vi "LOAD CELL READ.vi"(8 "error in (no error)":errorcluster, 11 "main ref":T1) -> (0 "error out":errorcluster)   [LabVIEW 2025]
uses:
  controls/LAB-IQ UI Data.ctl
  Traction Loop/Traction Receipe Enum.ctl
  v05/LOAD CELL CODE/New Logic/Load cell Enum.ctl
  <vilib>/Analysis/baseanly.llb/Mean (DBL).vi
  <vilib>/Analysis/5stat.llb/RMS (DBL).vi
  <vilib>/Analysis/Matrix/Numeric/Conversions/Array To Matrix - RA.vi
  <vilib>/Analysis/Matrix/Numeric/Conversions/Matrix To Array - RM.vi
  <vilib>/Analysis/NI_AALBase.lvlib
  <vilib>/ptbypt/NI_PtbyPt.lvlib
  <vilib>/Analysis/NI_AALPro.lvlib
  <vilib>/Analysis/Matrix/NI_Matrix.lvlib
panel:
  out "Fload 3":dbl
  out "Fload 2":dbl
  out "Fload":dbl
  out "Friction":dbl
  out "Load Temp":dbl
  out "Zload":dbl
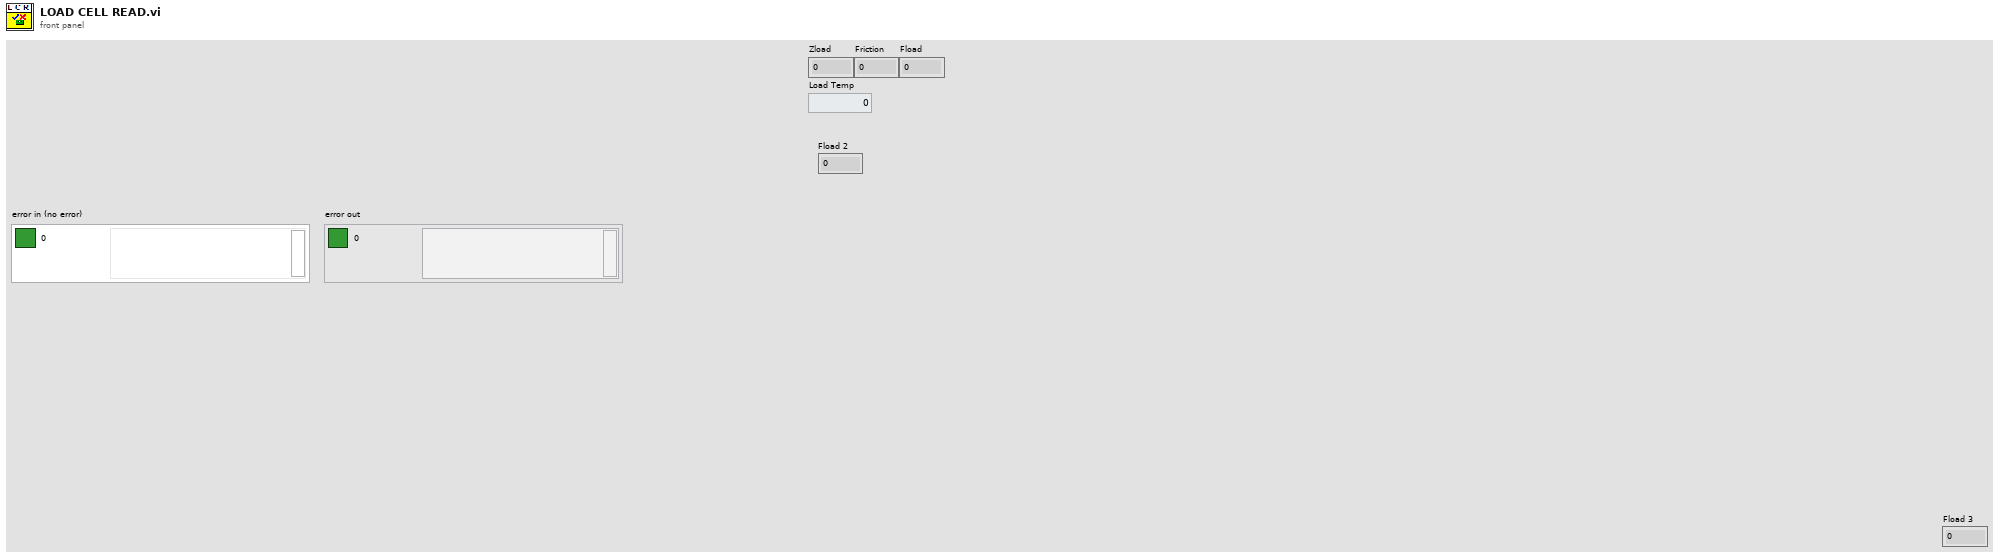
[diagram p1: front panel]
types:
  T1 = typedef "LAB-IQ UI Data.ctl" = cluster{"Main Home Screen":cluster{"GUI":refnum<vi>, "Platform Settings":refnum<vi>, "Configure":refnum<vi>, "Home":refnum<vi>, "EXIT":refnum<vi>, "service 2":refnum<vi>, "MainPage":refnum<vi>, "Analysis":refnum<vi>}, "Platform Settings":cluster{"mm/s  Surge":refnum<vi>, "Drive Error":refnum<vi>, "Disable Axis Jog Soft Limits":refnum<vi>, "mm/s  Sway":refnum<vi>, "Sway and Surge COM Status":refnum<vi>, "Heave COM Status":refnum<vi>, "Enable Platform":refnum<vi>, "Surge Forward Main":refnum<vi>, "Sway Right Main":refnum<vi>, "Sway Left Main":refnum<vi>, "Heave Down Main":refnum<vi>, "Heave Up main":refnum<vi>, "mm/s Heave":refnum<vi>, "mm/sec":refnum<vi>, "mm":refnum<vi>, "Surge Backward Main":refnum<vi>}, "Analysis Screen":cluster{"Analysis Home":refnum<vi>, "Surface Analysis":refnum<vi>, "Imaging":refnum<vi>, "Image Analysis":refnum<vi>, "Post Analysis":refnum<vi>}, "Config Screen":cluster{"Select Load Head":refnum<vi>, "Notes :":refnum<vi>, "FILE":refnum<vi>, "Sample ID :":refnum<vi>, "Operator ID :":refnum<vi>, "Operator Name :":refnum<vi>, "Auto":refnum<vi>}, "Motion Module":cluster{"zNL":refnum<vi>, "NL disp":refnum<vi>, "Rotary Tab":refnum<vi>, "Motion Direction:  3":refnum<vi>, "E.Velocity 2":refnum<vi>, "e.v/ssr 2":refnum<vi>, "Enter Fixed E.Velocity 2":refnum<vi>, "Enter Final SRR 2":refnum<vi>, "Enter initial SRR 2":refnum<vi>, "Enter Fixed SRR 2":refnum<vi>, "Enter the Final E.Velocity (m/s) 2":refnum<vi>, "Enter initial E.Velocity (m/s) 2":refnum<vi>, "Final Speed (RPM) 3":refnum<vi>, "Initial Speed (RPM) 2":refnum<vi>, "Enter the Final Velocity (m/s) 3":refnum<vi>, "Enter initial Velocity (m/s)  3":refnum<vi>, "Ramp Up 2":refnum<vi>, "TEST SELECTION":refnum<vi>, "SPEED SELECTION : ":refnum<vi>, "Angular Oscillation Set":refnum<vi>, "Traction":refnum<vi>, "Step Speed":refnum<vi>, "StepTable For Load-Speed":refnum<vi>, "StepTable For Speed":refnum<vi>, "Surge Forward MM":refnum<vi>, "Surge Backward MM":refnum<vi>, "M3 Image":refnum<vi>, "String 39":refnum<vi>, "Sway Left MM":refnum<vi>, "Sway Right MM":refnum<vi>, "Disable Axis Jog Soft Limits":refnum<vi>, "mm":refnum<vi>, "Heave Down MM":refnum<vi>, "Heave Up MM":refnum<vi>, "Wear Track Diameter (mm)":refnum<vi>, "Set WTD":refnum<vi>, "HomeScratch":refnum<vi>, "HomeRot":refnum<vi>, "PlaceModule":refnum<vi>, "Enter the Angle (Deg)":refnum<vi>, "Enter the Frequency (Hz)":refnum<vi>, "Motion Mode:":refnum<vi>, "LR Sway":refnum<vi>, "Rot Hor":refnum<vi>, "Scratch":refnum<vi>, "LR Cam":refnum<vi>, "MMBack":refnum<vi>, "MMNext":refnum<vi>, "Rot Ver":refnum<vi>, "Rotary Module Selection":refnum<vi>, "calculate rotary":refnum<vi>, "SPEED SELECTION : rotary":refnum<vi>, "Import 2":refnum<vi>, "Save 2":refnum<vi>, "File Path :  2":refnum<vi>, "String 45":refnum<vi>, "StepTable For Speed 3":refnum<vi>, "Enter the Speed(mm/sec)":refnum<vi>, "Enter the Speed(RPM)":refnum<vi>, "Enter Scratch Speed (mm/s):":refnum<vi>, "SwaySpeed Set":refnum<vi>, "Scartch Offset":refnum<vi>, "Motion type:":refnum<vi>, "HomeScratch 2":refnum<vi>, "Enter Scratch length (mm):":refnum<vi>, "Wear Track Diameter":refnum<vi>, "Rotary Speed Exced":refnum<vi>, "Scratch Mode":refnum<vi>, "No of Scratch":refnum<vi>}, "Environmental control":cluster{"Humidity  Status  3":refnum<vi>, "Low Temp  Status  2":refnum<vi>, "TK4 status 2":refnum<vi>, "Stage Temperature":refnum<vi>, "Sample Temperature":refnum<vi>, "Humidity (Amb)":refnum<vi>, "Clear List":refnum<vi>, "Add to list":refnum<vi>, "Wear":refnum<vi>, "Vibration":refnum<vi>, "Humidity (Chamber)":refnum<vi>, "Temperature (Chamber)":refnum<vi>, "ECR ":refnum<vi>, "Temperature (Amb)":refnum<vi>, "Microphone":refnum<vi>, "Acoustic Emission 3":refnum<vi>, "SNext":refnum<vi>, "APBack":refnum<vi>, "Enter the Temperature (°C):":refnum<vi>, "Enter the Stage \nTemperature (°C):":refnum<vi>, "Enter the Humidity (%Rh):":refnum<vi>, "Low Temp":refnum<vi>, "High Temp":refnum<vi>, "Humidity":refnum<vi>, "Sensors Picked":refnum<vi>}, "About Screen":cluster{"Password":refnum<vi>, "Home Service":refnum<vi>, "Advanced Setting":refnum<vi>, "About Tab":refnum<vi>, "ECR Port:":refnum<vi>, "Ramp Port:":refnum<vi>, "Installation/Replacement completed":refnum<vi>, "Loahead":refnum<vi>, "Heave and Surge COM Port:":refnum<vi>, "Sway COM Port:":refnum<vi>, "Temp Modbus:":refnum<vi>, "Humidity Port:":refnum<vi>, "Edit Gain Constants":refnum<vi>, "Save Gain Constants":refnum<vi>}, "Main Screen":cluster{"Main Screen Tab":refnum<vi>, "Angle and Frequency":refnum<vi>, "Stroke (mm)":refnum<vi>, "Angle (Deg)":refnum<vi>, "Main Speed Tab":refnum<vi>, "MTM MOTOR DISPLAY":refnum<vi>, "Disc Speed (m/sec)":refnum<vi>, "Ball Speed (m/sec)":refnum<vi>, "Disc Speed (RPM)":refnum<vi>, "Ball Speed (RPM)":refnum<vi>, "SPEED TAB":refnum<vi>, "Speed (m/sec)":refnum<vi>, "Set Speed (m/sec)":refnum<vi>, "Speed (RPM)":refnum<vi>, "Set Speed":refnum<vi>, "Time Tab":refnum<vi>, "Time ( HH:MM:SS ) 2":refnum<vi>, "Test Duration":refnum<vi>, "Test Duration 4":refnum<vi>, "TEST CYCLE":refnum<vi>, "TOTAL CYCLES":refnum<vi>, "Set Load (N)":refnum<vi>, "Temp Tabs":refnum<vi>, "Heater":refnum<vi>, "TK4 status":refnum<vi>, "ChamberTemp":refnum<vi>, "SetTmp":refnum<vi>, "Controller  Status":refnum<vi>, "ChamberTemp 2":refnum<vi>, "SetTmp 2":refnum<vi>, "Controller  Status 2":refnum<vi>, "ChamberTemp 3":refnum<vi>, "SetTmp 3":refnum<vi>, "Cooling":refnum<vi>, "Load Communication":refnum<vi>, "Ambient \nTemperature":refnum<vi>, "HumCOMStatus":refnum<vi>, "Ambient\n Humidity":refnum<vi>, "Freq (Hz)":refnum<vi>, "Load En":refnum<vi>, "NLt":refnum<vi>, "zNL 2":refnum<vi>, "Humidity On":refnum<vi>, "humidity disp":refnum<vi>, "Set Humidity":refnum<vi>, "NL disp 2":refnum<vi>, "Humidity On 2":refnum<vi>, "humidity disp 2":refnum<vi>, "Set Humidity 2":refnum<vi>, "NL disp 3":refnum<vi>, "AppLoadSeq scratch":refnum<vi>, "Stop Scratch":refnum<vi>, "ClrLog":refnum<vi>, "Trip Log":refnum<vi>, "STOP":refnum<vi>, "Start Test":refnum<vi>, "Test status":refnum<vi>, "AR Led":refnum<vi>, "Data":refnum<vi>, "Health":refnum<vi>, "Sway COM Status":refnum<vi>, "Heave COM Status":refnum<vi>, "Grp Tab":refnum<vi>, "Sub Graph":refnum<vi>, "SD (mm)":refnum<vi>, "Siliding distance Reset Graph":refnum<vi>, "SDGp":refnum<vi>, "Humidity Reset Graph":refnum<vi>, "HumrGp":refnum<vi>, "Acoustic Emission (mV)":refnum<vi>, "Aqucostic Reset Graph":refnum<vi>, "gACQUOS":refnum<vi>, "ECR RESET":refnum<vi>, "ECR":refnum<vi>, "Temperature Reset":refnum<vi>, "Acoustic Emission (mV) 2":refnum<vi>, "Aqucostic Reset Graph 2":refnum<vi>, "gACQUOS 2":refnum<vi>, "ECR RESET 2":refnum<vi>, "ECR 2":refnum<vi>, "Temperature Reset 2":refnum<vi>, "Temperature (deg c)":refnum<vi>, "Speed Reset Graph":refnum<vi>, "Speed Tab":refnum<vi>, "MTM DISC  SPEED":refnum<vi>, "MTM BALL SPEED":refnum<vi>, "speed mm/sec":refnum<vi>, "Hymidity":refnum<vi>, "Humidity Disable trip":refnum<vi>, "CoF Trip  2":refnum<vi>, "Depth Trip":refnum<vi>, "Weart Deapth":refnum<vi>, "Depth Reset Graph":refnum<vi>, "Weart":refnum<vi>, "Depthz":refnum<vi>, "Depth (µm)":refnum<vi>, "WearGp":refnum<vi>, "NL Trip 2":refnum<vi>, "Load pid":refnum<vi>, "Load Disable Trip":refnum<vi>, "Load Reset Graph":refnum<vi>, "NL Display 4":refnum<vi>, "Main Chart 3":refnum<vi>, "BACK":refnum<vi>, "Depth Trip 2":refnum<vi>, "COF TRIP ":refnum<vi>, "Friction Force (N)":refnum<vi>, "FF Reset Graph":refnum<vi>, "FF Disable Trip":refnum<vi>, "FF TRIP":refnum<vi>, "COF Disable Trip":refnum<vi>, "COF Reset Graph":refnum<vi>, "Start Test Temp":refnum<vi>, "zFF":refnum<vi>, "Friction Force (N) Graph":refnum<vi>, "Coefficient of Friction":refnum<vi>, "Scratch Start Test":refnum<vi>, "FF Tab":refnum<vi>, "Cyclic Friction Force (N)":refnum<vi>, "CZ FF":refnum<vi>, "Cyclic Friction Force (N) Graph":refnum<vi>, "Cyclic Coefficient of Friction":refnum<vi>, "Cyclic FF TRIP":refnum<vi>, "Cyclic FF Disable Trip":refnum<vi>, "cyclic COF Disable Trip":refnum<vi>, "cyclic COF TRIP":refnum<vi>, "cyclic COF Reset Graph":refnum<vi>, "Cyclic FF Reset Graph":refnum<vi>, "Test Trip":refnum<vi>, "Multi Scratch Pass":refnum<vi>, "Scratch Start Recording":refnum<vi>}, "Loading":cluster{"Indentation":refnum<vi>, "Reference Sample":refnum<vi>, "Load Cell Communication Slide":refnum<vi>, "com 3":refnum<vi>, "com":refnum<vi>, "DecaForce COM Status":refnum<vi>, "Update":refnum<vi>, "Clear 3":refnum<vi>, "seq":refnum<vi>, "Stribeck table":refnum<vi>, "Stribeck Table  For loading":refnum<vi>, "Loading Mode":refnum<vi>, "Enter the Final Load (N)":refnum<vi>, "Enter the CoF Trip":refnum<vi>, "Enter the Friction Force Trip":refnum<vi>, "Enter the Normal load Trip":refnum<vi>, "Enter the Load  (N)":refnum<vi>, "KiloForce":refnum<vi>, "DecaForce ":refnum<vi>, "MicroForce":refnum<vi>, "LHBack":refnum<vi>, "LHNext":refnum<vi>, "Enter the Loading Rate (N/min)":refnum<vi>, "Message":refnum<vi>, "Warning 2":refnum<vi>, "SSP 0.75":refnum<vi>, "SSP 0.5":refnum<vi>, "SSP 0.3":refnum<vi>, "Warning":refnum<vi>, "gui GIF":refnum<vi>, "Communication is established":refnum<vi>, "AppLoad 4":refnum<vi>, "Multipoint":refnum<vi>, "Load Selection":refnum<vi>}, "PID":cluster{"Ramp":refnum<vi>, "Vertical load (N)":refnum<vi>, "apply load":refnum<vi>, "apply load 2":refnum<vi>, "Enter ByPass Load":refnum<vi>, "Bypass Load":refnum<vi>, "gFF Rot":refnum<vi>}, "Config Parameters":cluster{"Tab Control 3":refnum<vi>, "Tab Control 19":refnum<vi>, "SAMPLES":refnum<vi>, "Re-initilaize":refnum<vi>, "Filter ON/OFF":refnum<vi>, "TracHomeSurgeOffsetCounts 10MM":refnum<vi>, "TracHomeSwayOffsetCounts 10MM":refnum<vi>, "Acoustic Emission:":refnum<vi>, "Apply Filter (FF)":refnum<vi>, "Filter% 2":refnum<vi>, "Apply Filter (Load)":refnum<vi>, "Filter% ":refnum<vi>, "Sway distance (mm)":refnum<vi>, "Surge distance (mm)":refnum<vi>, "DataSavingLoopDelay(ms)":refnum<vi>, "SAVE 2":refnum<vi>, "Enter Distance":refnum<vi>, "Sway Counts:":refnum<vi>, "Distance (mm): 3":refnum<vi>, "Surge Counts:":refnum<vi>, "Distance (mm): 2":refnum<vi>, "Distance (mm):":refnum<vi>, "Heave Counts:":refnum<vi>, "LRMHomeSurgeOffsetCounts":refnum<vi>, "LRMHomeSwayOffsetCounts":refnum<vi>, "TracHomeSurgeOffsetCounts 20MM":refnum<vi>, "TracHomeSwayOffsetCounts 20MM":refnum<vi>, "RotHomeSwayOffsetCounts":refnum<vi>, "RotHomeSurgeOffsetCounts":refnum<vi>, "Heave distance":refnum<vi>, "Zmm":refnum<vi>, "Heave Pulses/mm":refnum<vi>, "Surge Pulses/mm":refnum<vi>, "Sway Pulses/mm":refnum<vi>, "Heave Pitch":refnum<vi>, "Surge Pitch":refnum<vi>, "Sway Pitch":refnum<vi>, "Heave PPR":refnum<vi>, "Surge PPR":refnum<vi>, "Sway PPR":refnum<vi>, "Tab Control 5":refnum<vi>, "Tab Control 14":refnum<vi>, "Tab Control 26":refnum<vi>, "AE":refnum<vi>, "Heave Loop Delay":refnum<vi>, "Heave PID Speed":refnum<vi>, "Surge Jog Speed":refnum<vi>, "Heave Jog Speed":refnum<vi>, "Sway Loop Delay":refnum<vi>, "Sway PID Speed":refnum<vi>, "Sway Jog Speed":refnum<vi>, "DEPTH TRIP VALUE":refnum<vi>, "LOAD TRIP VALUE":refnum<vi>, "DEPTH TRIP   ENABLE":refnum<vi>, "LOAD TRIP  ENABLE":refnum<vi>, "CYCLIC FF TRIP VALUE":refnum<vi>, "FF TRIP VALUE":refnum<vi>, "CYCLIC CoF TRIP VALUE":refnum<vi>, "COF TRIP VALUE":refnum<vi>, "CYCLIC COF TRIP  ENABLE":refnum<vi>, "CYCLIC FF TRIP  ENABLE":refnum<vi>, "FF TRIP  ENABLE":refnum<vi>, "COF TRIP  ENABLE":refnum<vi>, "JOG TRIP LOAD VALUE (N)":refnum<vi>, "Rotary Vertical":refnum<vi>, "Traction":refnum<vi>, "Scratch":refnum<vi>, "LRM CAM":refnum<vi>, "Sway LRM":refnum<vi>, "Rotary Horizontal":refnum<vi>}, "Loading Com Port":cluster{"ClearAll":refnum<vi>, "Mz(Nm)":refnum<vi>, "My(Nm)":refnum<vi>, "Mx(Nm)":refnum<vi>, "Save Dwell":refnum<vi>, "Acq Delay (ms)":refnum<vi>, "Burst Delay (ms)":refnum<vi>, "model":refnum<vi>, "SN":refnum<vi>, "FFx(N)":refnum<vi>, "Sensor IP":refnum<vi>, "Port":refnum<vi>, "FFy(N)":refnum<vi>, "Load(N)":refnum<vi>, "delete Handle":refnum<vi>, "Create Handle":refnum<vi>, "ft_data":refnum<vi>, "ft_range":refnum<vi>, "ft_data 2":refnum<vi>, "stop 6":refnum<vi>, "running_flag":refnum<vi>, "ft_udp_handle":refnum<vi>, "get-data-return":refnum<vi>, "get-range-return":refnum<vi>, "zero-return":refnum<vi>, "filter-return":refnum<vi>, "initial-return":refnum<vi>, "deleteHandle-result":refnum<vi>, "Load Cell Temp":refnum<vi>, "Load Cell":refnum<vi>, "ZeroAll":refnum<vi>, "FORCE (N)":refnum<vi>, "TORQUE (N-m)":refnum<vi>, "Load Cell Link":refnum<vi>}, "Heave AND Surge":cluster{"SURGE POSE":refnum<vi>, "error out Read":refnum<vi>, "HEAVE POSE":refnum<vi>, "State":refnum<vi>, "Homed":refnum<vi>, "Sequence ID":refnum<vi>, "error out Write":refnum<vi>, "faultCode":refnum<vi>, "Ack ID":refnum<vi>, "SPEED":refnum<vi>, "Distance":refnum<vi>, "Mode Command":refnum<vi>, "Heave and Surge Read":refnum<vi>, "Read Heave Temp":refnum<vi>, "Spare 15":refnum<vi>, "Spare 14":refnum<vi>, "Spare 13":refnum<vi>, "Spare 12":refnum<vi>, "Spare 11":refnum<vi>, "Spare 10":refnum<vi>, "Spare 9":refnum<vi>, "Spare 8":refnum<vi>, "Spare 7":refnum<vi>, "Spare 4":refnum<vi>, "Spare 3":refnum<vi>, "Spare 2":refnum<vi>, "Humidity":refnum<vi>, "Temp":refnum<vi>, "Node Id":refnum<vi>, "Spare 1":refnum<vi>, "SPARE 4":refnum<vi>, "SPARE 3":refnum<vi>, "SPARE 2":refnum<vi>, "SPARE 1":refnum<vi>, "fwMajor":refnum<vi>, "fwMinor":refnum<vi>, "Manual Write":refnum<vi>, "Heave and Surge Write":refnum<vi>, "SPARE 5":refnum<vi>, "Reserved ":refnum<vi>, "SPARE 8":refnum<vi>, "SPARE 6":refnum<vi>, "SPARE 7":refnum<vi>, "SPARE 17":refnum<vi>, "SPARE 16":refnum<vi>, "SPARE 15":refnum<vi>, "SPARE 14":refnum<vi>, "SPARE 13":refnum<vi>, "SPARE 12":refnum<vi>, "SPARE 11":refnum<vi>, "SPARE 10":refnum<vi>, "SPARE 9":refnum<vi>, "System UPTIME":refnum<vi>, "Missed Packets":refnum<vi>, "faultCode Surge Right":refnum<vi>, "faultCode Surge Left":refnum<vi>, "faultCode Heave":refnum<vi>, "UPLINK HEAVE":refnum<vi>, "DOWNLINK HEAVE":refnum<vi>}, "New PID LOGIC":cluster{"Fine Tune Zone":refnum<vi>, "PID SDelay":refnum<vi>, "Max_pos_limit":refnum<vi>, "Min_pos_limit":refnum<vi>, "i_limit":refnum<vi>, "pct_scale":refnum<vi>, "Deadband":refnum<vi>, "Kd":refnum<vi>, "Ki":refnum<vi>, "Kp":refnum<vi>, "Current Position":refnum<vi>, "Set Load":refnum<vi>, "Current Load":refnum<vi>, "Pulse delta":refnum<vi>, "Init Step":refnum<vi>, "Max Step Linit":refnum<vi>, "min_deadband_floor":refnum<vi>, "dynamic_spindle_noise_scalar":refnum<vi>, "min_finetune_floor":refnum<vi>, "filter_alpha":refnum<vi>, "PID":refnum<vi>}, "SWAY ":cluster{"fwMajor":refnum<vi>, "Homed":refnum<vi>, "Rotary POSE":refnum<vi>, "State":refnum<vi>, "SWAY POSE":refnum<vi>, "Ack ID":refnum<vi>, "faultCode":refnum<vi>, "Node Id":refnum<vi>, "fwMinor":refnum<vi>, "Spare 6":refnum<vi>, "Spare 5":refnum<vi>, "Spare 4":refnum<vi>, "Spare 3":refnum<vi>, "Spare 2":refnum<vi>, "Spare 1":refnum<vi>, "Spare 7":refnum<vi>, "SPARE  5":refnum<vi>, "error out Write  SWAY ":refnum<vi>, "error out Read SWAY ":refnum<vi>, "Manual Write SWAY ":refnum<vi>, "SWAY WRITE":refnum<vi>, "SPARE  4":refnum<vi>, "SPARE  3":refnum<vi>, "SPARE 2":refnum<vi>, "SPARE 1":refnum<vi>, "Spare 15":refnum<vi>, "Spare 14":refnum<vi>, "Spare 13":refnum<vi>, "Spare 12":refnum<vi>, "Spare 11":refnum<vi>, "Spare 9":refnum<vi>, "Spare 8":refnum<vi>, "SPEED":refnum<vi>, "Distance":refnum<vi>, "Mode Command":refnum<vi>, "Sequence ID":refnum<vi>, "SWAY READ":refnum<vi>, "Spare 10":refnum<vi>, "Read SWAY Temp":refnum<vi>, "faultCode Sway ":refnum<vi>, "Missed Packets":refnum<vi>, "System UPTIME sway":refnum<vi>, "SPARE 6":refnum<vi>, "SPARE 7":refnum<vi>, "SPARE 9":refnum<vi>, "SPARE 11":refnum<vi>, "SPARE 10":refnum<vi>, "SPARE 8":refnum<vi>, "SPARE 13":refnum<vi>, "SPARE 12":refnum<vi>, "SPARE 17":refnum<vi>, "SPARE 16":refnum<vi>, "SPARE 15":refnum<vi>, "SPARE 14":refnum<vi>, "Reserved":refnum<vi>, "faultCode Rotary":refnum<vi>, "UPLINK SWAY":refnum<vi>, "DOWNLINK SWAY":refnum<vi>}, "Analysis Screen":cluster{"Analysis Home":refnum<vi>, "Refresh 2":refnum<vi>, "MEAN 4":refnum<vi>, "SD 4":refnum<vi>, "VARIANCE 4":refnum<vi>, "MEAN  3":refnum<vi>, "SD  3":refnum<vi>, "VARIANCE  3":refnum<vi>, "MEAN 2":refnum<vi>, "SD  2":refnum<vi>, "VARIANCE 2":refnum<vi>, "MEAN":refnum<vi>, "SD":refnum<vi>, "VARIANCE":refnum<vi>, "File 4 Discription":refnum<vi>, "OPEN 4":refnum<vi>, "File Name 4":refnum<vi>, "OPEN 3":refnum<vi>, "File 3 Discription":refnum<vi>, "File Name 3":refnum<vi>, "Y-AXIS":refnum<vi>, "X-AXIS":refnum<vi>, "XY Graph":refnum<vi>, "File Name 2":refnum<vi>, "File Name 1":refnum<vi>, "OPEN 2":refnum<vi>, "OPEN 1":refnum<vi>, "File 1 Discription ":refnum<vi>, "File 2 Discription":refnum<vi>, "Export":refnum<vi>, "File Format":refnum<vi>}, "Traction":cluster{"faultCode Traction 2":refnum<vi>, "faultCode Traction 1":refnum<vi>, "Missed Packets":refnum<vi>, "System UPTIME Traction":refnum<vi>, "SPARE 17":refnum<vi>, "SPARE 16":refnum<vi>, "SPARE 15":refnum<vi>, "SPARE 14":refnum<vi>, "SPARE 13":refnum<vi>, "SPARE 12":refnum<vi>, "SPARE 11":refnum<vi>, "SPARE 10":refnum<vi>, "SPARE 9":refnum<vi>, "SPARE 8":refnum<vi>, "SPARE 7":refnum<vi>, "SPARE 6":refnum<vi>, "Reserved":refnum<vi>, "SPARE  5":refnum<vi>, "Manual Write TRACTION":refnum<vi>, "TRACTION WRITE":refnum<vi>, "SPARE  4":refnum<vi>, "SPARE  3":refnum<vi>, "SPARE 2":refnum<vi>, "SPARE 1":refnum<vi>, "Spare 7":refnum<vi>, "Spare 6":refnum<vi>, "Spare 5":refnum<vi>, "Spare 4":refnum<vi>, "Spare 2":refnum<vi>, "Spare 1":refnum<vi>, "Node Id":refnum<vi>, "Read TRACTION Temp":refnum<vi>, "fwMinor":refnum<vi>, "fwMajor":refnum<vi>, "faultCode":refnum<vi>, "TRACTION POSE":refnum<vi>, "TRACTION POSE 2":refnum<vi>, "Homed":refnum<vi>, "State":refnum<vi>, "Ack ID":refnum<vi>, "SPEED":refnum<vi>, "Distance":refnum<vi>, "Mode Command":refnum<vi>, "Sequence ID":refnum<vi>, "error out Read TRACTION":refnum<vi>, "error out Write  TRACTION":refnum<vi>, "TRACTION READ":refnum<vi>, "Spare 3":refnum<vi>, "Downlink traction":refnum<vi>, "Uplink Traction":refnum<vi>}, "Traction reciepe":cluster{"SRR Sweep Range (%) Stribeck":refnum<vi>, "Traction Receipe":refnum<vi>, "Total Execution Time":refnum<vi>, "Total Steps":refnum<vi>, "Duration / Step (s)  Stribeck":refnum<vi>, "STRIBECK Fixed SRR List (%)":refnum<vi>, "Duration / Step (s) Traction":refnum<vi>, "SRR Sweep Range (%) traction":refnum<vi>, "Rolling Speed (mm/s)":refnum<vi>, "Temperature Stages (°C)":refnum<vi>, "Ball Load (N)":refnum<vi>, "Lubricant Name":refnum<vi>, "Profile File Name":refnum<vi>, "SET entrainment Velocity":refnum<vi>, "Test Array Size":refnum<vi>, "SRR INDEX [ STRIBECK]":refnum<vi>, "Stribeck Size":refnum<vi>, "SET SRR":refnum<vi>, "ELAPSED TIMER ":refnum<vi>, "BALL SET RPM":refnum<vi>, "DISC SET RPM":refnum<vi>, "SET LOAD":refnum<vi>, "TEMPERATURE READ":refnum<vi>, "SET TEMPERATURE":refnum<vi>, "Traction Size":refnum<vi>, "DISC SPEED (rpm)":refnum<vi>, "BALL SPEED (rpm)":refnum<vi>, "BALL WEAR TRACK":refnum<vi>, "DISC WEARTRACK":refnum<vi>, "SRR INDEX [ TRACTION]":refnum<vi>, "Start Index Type":refnum<vi>, "Enum - Menu":refnum<vi>, "Ball (mm/sec)":refnum<vi>, "Disc (mm/sec)":refnum<vi>}, "Traction Control":cluster{"HomeTraction":refnum<vi>, "Demo Mode Display":refnum<vi>, "Traction Message":refnum<vi>, "Traction Step Update Details":refnum<vi>, "Main Tab sequence for selection":refnum<vi>, "Ramp Tab":refnum<vi>, "e.v/ssr":refnum<vi>, "Enter Fixed E.Velocity":refnum<vi>, "Enter Final SRR":refnum<vi>, "Enter initial SRR":refnum<vi>, "Enter Fixed SRR":refnum<vi>, "Enter the Final E.Velocity (m/s)":refnum<vi>, "Enter initial E.Velocity (m/s)":refnum<vi>, "Ball WTD":refnum<vi>, "E.Velocity":refnum<vi>, "Enter the Final Velocity (m/s)":refnum<vi>, "Enter initial Velocity (m/s)":refnum<vi>, "Ramp Up   Disc":refnum<vi>, "Initial DiscSpeed (RPM)":refnum<vi>, "Final Speed (RPM) Ball":refnum<vi>, "Final Speed (RPM)":refnum<vi>, "Initial Speed (RPM) Ball":refnum<vi>, "Enter the Final Velocity (m/s) Ball":refnum<vi>, "Enter initial Velocity (m/s) Ball":refnum<vi>, "Ramp Up":refnum<vi>, "ExceedBallSpeed step":refnum<vi>, "ExceedDiscSpeed":refnum<vi>, "BallSpeed Exceed Indication":refnum<vi>, "Apply":refnum<vi>, "SPEED SELECTION : MTM":refnum<vi>, "SPEED SELECTION : MTM 2":refnum<vi>, "TEST SELECTION (MTM)":refnum<vi>, "MTM Test Selection":refnum<vi>, "File Path Tab":refnum<vi>, "File Path String":refnum<vi>, "Save":refnum<vi>, "Save  2":refnum<vi>, "Import ":refnum<vi>, "File Path :":refnum<vi>, "Step Sequence Indication Tab":refnum<vi>, "Step Sequence Indication":refnum<vi>, "Calculate Step":refnum<vi>, "StepTable":refnum<vi>, "ExceedDiscSpeed  Cinstant Speed":refnum<vi>, "ExceedBallSpeed Constant":refnum<vi>, "TEST SELECTION (MTM) 2":refnum<vi>, "SPEED SELECTION : MTM 3":refnum<vi>, "MTM Test Selection 2":refnum<vi>, "Enter the Speed (m/sec): ":refnum<vi>, "Enter the Speed (m/sec):  2":refnum<vi>, "Enter the Speed (RPM):":refnum<vi>, "Lower Spped ":refnum<vi>, "Upper":refnum<vi>, "Enter the Speed (RPM):Ball":refnum<vi>, "Disc Motion Direction: ":refnum<vi>, "Ball Motion Direction :":refnum<vi>, "Motion Mode: ":refnum<vi>, "Wear Track Diameter (mm) ":refnum<vi>, "Disc Speed Indicator":refnum<vi>, "ExceedBallSpeed":refnum<vi>}, "Acquostic":cluster{"Last Config Rejected ":refnum<vi>, "rx command count":refnum<vi>, "Current Filter Id":refnum<vi>, "Isolated Gain":refnum<vi>, "DAQ Status":refnum<vi>, "error out":refnum<vi>, "error in (no error)":refnum<vi>, "Uplink Packet":refnum<vi>, "data out":refnum<vi>, "Downlink Packet":refnum<vi>, "Gains":refnum<vi>, "Manual Write Acquostic":refnum<vi>, "Acoustic Graphs":refnum<vi>}}
  T2 = cluster{"model":string, "SN":i32, "Sensor IP":string, "Port":i32, "Acq Delay (ms)":dbl, "Burst Delay (ms)":dbl, "Save Dwell":dbl, "FORCE (N)":dbl[][], "TORQUE (N-m)":dbl[][], "ft_data":dbl[], "running_flag":bool, "ClearAll":bool, "ZeroAll":bool}
  T3 = typedef "Load cell Enum.ctl" = enum16{"Init", "set UDP", "Read Info", "set Low Pass Filter", "Set Zero", "get data", "close", "REInit"}
  T4 = typedef "NI_Matrix.lvlib/RealMatrix.ctl" = dbl[][]
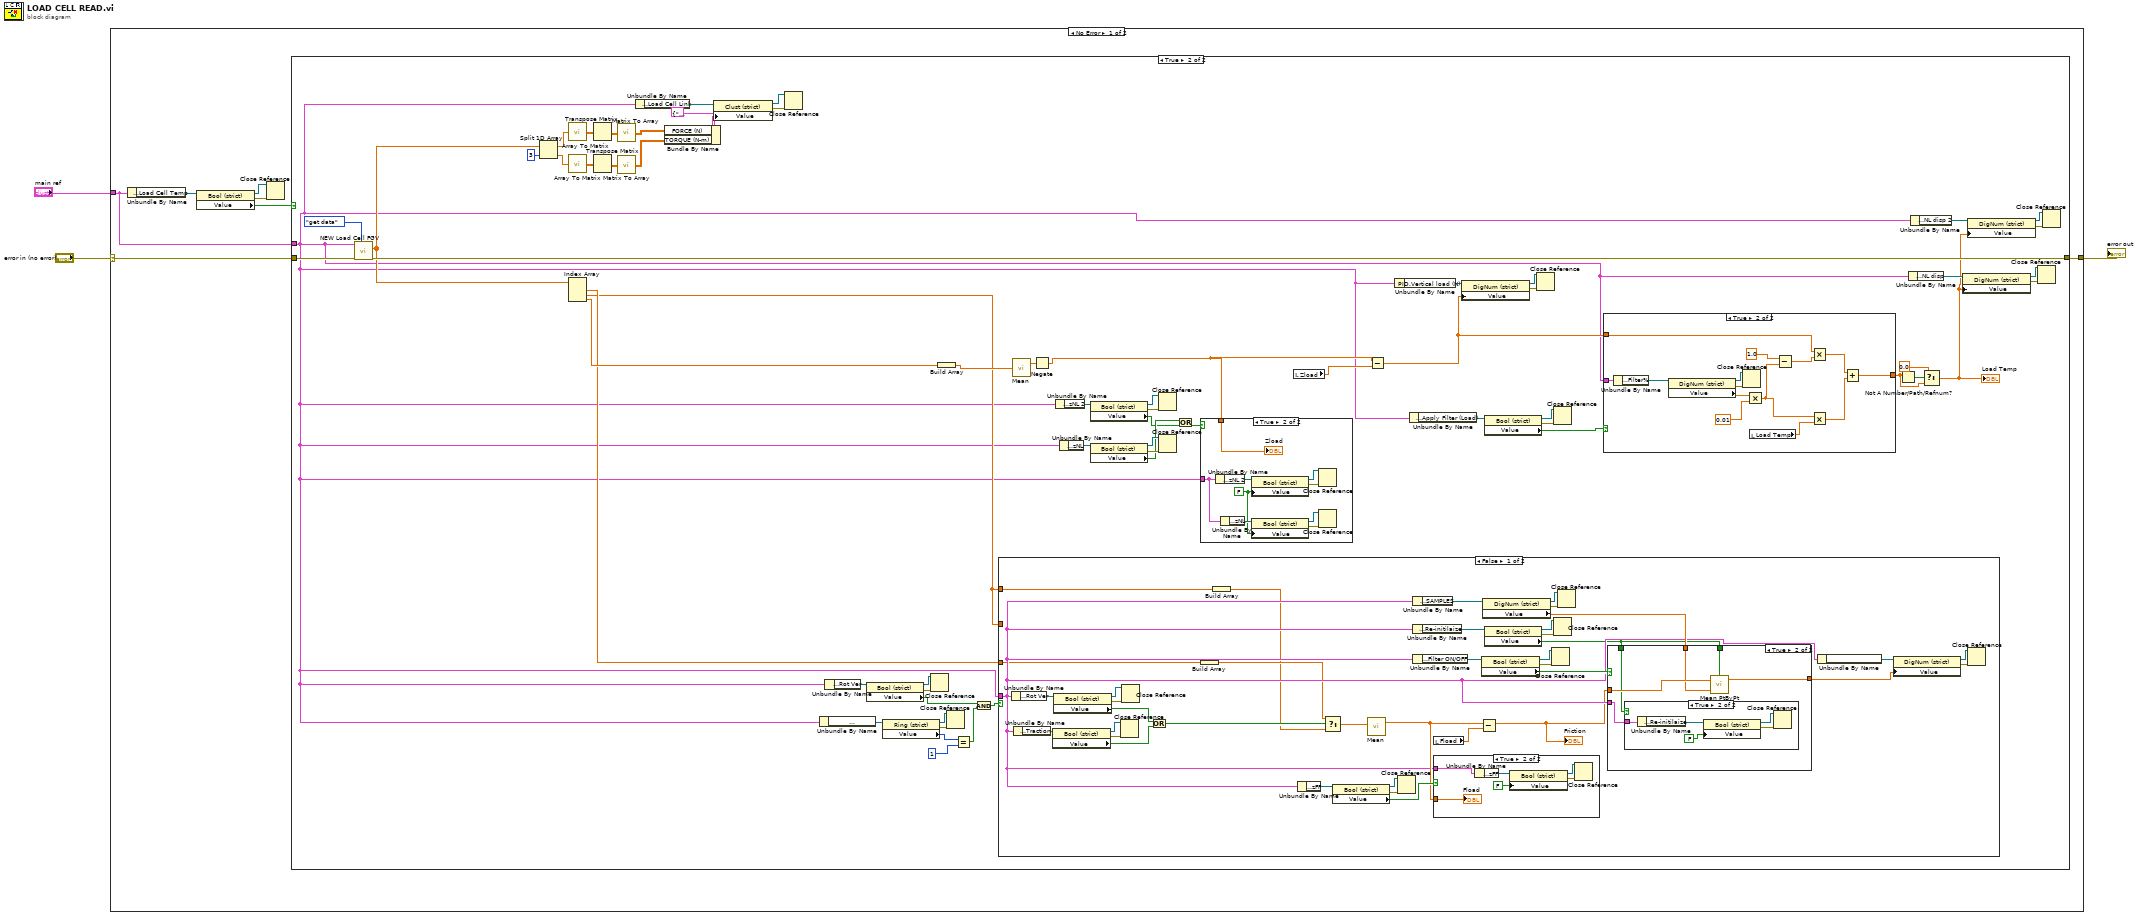
[diagram p0: block diagram]
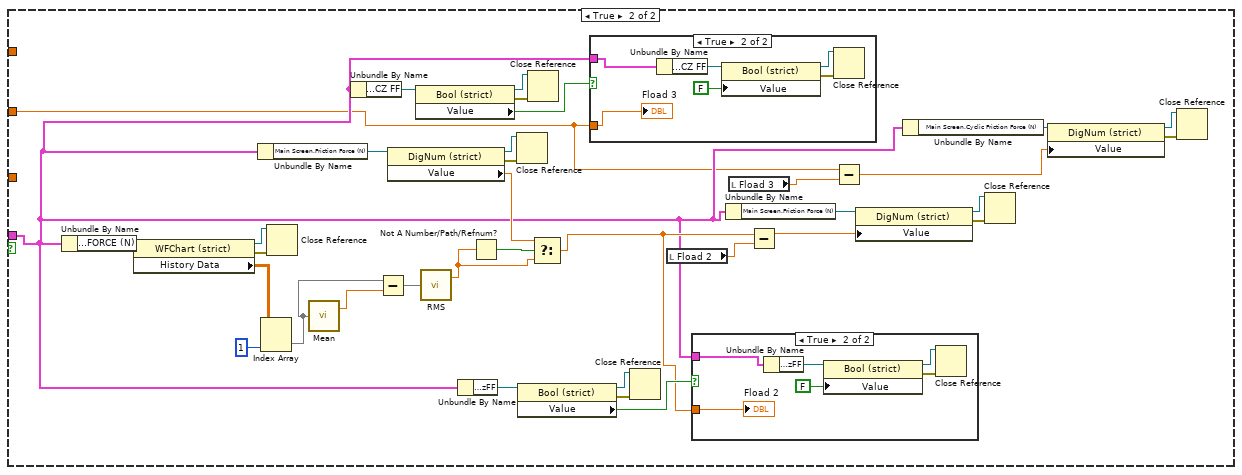
[diagram p6: hidden frame]
diagram:
  n1 = case shown="No Error" "error in (no error)" {
    selector: "error in (no error)" -> [w6 _]
    tunnel: "main ref" -> [w4 _]
    tunnel: [w5 _] -> w1
    frame No Error {
      n2 = Unbundle By Name(w4) -> ("Loading Com Port.Load Cell Temp"=w8:refnum<vi>)
      n3 = property class="Bool (strict)"(reference=w8) -> (reference out=w10:refnum<vi>, error out=w9:errorcluster, "Value"=w7:bool)  [unwired: 1 in]
      n4 = Close Reference(reference=w10, error in (no error)=w9) -> ()  [unwired: 1 out]
      n5 = case shown="True" w7 {
        tunnel: w6 -> [w11 w75]
        tunnel: [w11 w74] -> w5
        tunnel: w4 -> [_ w14]
        frame False {
        }
        frame True {
          n6 = call "NEW Load Cell FGV.vi"("Enum - Menu"=Load_cell_Enum."get data", "error in (no error)"=w75, "main ref"=w14) -> ("error out"=w74:errorcluster, "FT Data"=w22:dbl[])  [unwired: 7 in]
          n7 = Split 1D Array(array=w22, index=3) -> (first subarray=w29:dbl[], second subarray=w26:dbl[])
          n8 = call-poly <vilib>:"Array To Matrix.vi"("Real 1D Array"=w29) -> ("Real Matrix (Column Vector)"=w31:T4)
          n9 = call-poly <vilib>:"Array To Matrix.vi"("Real 1D Array"=w26) -> ("Real Matrix (Column Vector)"=w28:T4)
          n10 = Index Array(array=w22) -> (element #1=w21:dbl, element #2=w20:dbl, element #3=w25:dbl)  [unwired: 3 in]
          n11 = Transpose Matrix(1:w31) -> (0:w30:T4)
          n12 = Transpose Matrix(1:w28) -> (0:w27:T4)
          n13 = call-poly <vilib>:"Matrix To Array.vi"("Real Matrix"=w30) -> ("Real 2D Array"=w13:dbl[][])
          n14 = call-poly <vilib>:"Matrix To Array.vi"("Real Matrix"=w27) -> ("Real 2D Array"=w12:dbl[][])
          n15 = Unbundle By Name(w14) -> ("Loading Com Port.Load Cell Link"=w19:refnum<vi>)
          n16 = Bundle By Name(cluster=T2 {"model"="", "SN"=0, "Sensor IP"="", "Port"=0, "Acq Delay (ms)"=0.0, "Burst Delay (ms)"=0.0, "Save Dwell"=0.0, "FORCE (N)"=[], "TORQUE (N-m)"=[], "ft_data"=[], "running_flag"=FALSE, "ClearAll"=FALSE, "ZeroAll"=FALSE} ("Value"), "FORCE (N)"=w13, "TORQUE (N-m)"=w12) -> (w15:T2)
          n17 = property class="Clust (strict)"(reference=w19, "Value"=w15) -> (reference out=w17:refnum<vi>, error out=w18:errorcluster)  [unwired: 1 in]
          n18 = Close Reference(reference=w17, error in (no error)=w18) -> ()  [unwired: 1 out]
          n19 = Unbundle By Name(w14) -> ("Motion Module.Motion Mode:"=w38:refnum<vi>)
          n20 = Unbundle By Name(w14) -> ("Motion Module.Rot Ver"=w43:refnum<vi>)
          n21 = property class="Bool (strict)"(reference=w43) -> (reference out=w41:refnum<vi>, error out=w42:errorcluster, "Value"=w35:bool)  [unwired: 1 in]
          n22 = property class="Ring (strict)"(reference=w38) -> (reference out=w40:refnum<vi>, error out=w39:errorcluster, "Value"=w37:u16)  [unwired: 1 in]
          n23 = Close Reference(reference=w41, error in (no error)=w42) -> ()  [unwired: 1 out]
          n24 = Build Array(w25) -> (w24:dbl[])
          n25 = Close Reference(reference=w40, error in (no error)=w39) -> ()  [unwired: 1 out]
          n26 = Equal?(x=w37, y=u16 1) -> (x = y?=w34:bool)
          n27 = And(x=w35, y=w34) -> (x .and. y?=w33:bool)
          n28 = case shown="False" w33 {
            tunnel: w14 -> [w84 w138]
            tunnel: w20 -> [_ w132]
            tunnel: w21 -> [w79 _]
            tunnel: w20 -> [w78 _]
            frame False {
              n29 = Unbundle By Name(w84) -> ("Motion Module.Rot Ver"=w106:refnum<vi>)
              n30 = Unbundle By Name(w84) -> ("Motion Module.Traction"=w111:refnum<vi>)
              n31 = property class="Bool (strict)"(reference=w111) -> (reference out=w109:refnum<vi>, error out=w110:errorcluster, "Value"=w113:bool)  [unwired: 1 in]
              n32 = property class="Bool (strict)"(reference=w106) -> (reference out=w108:refnum<vi>, error out=w107:errorcluster, "Value"=w112:bool)  [unwired: 1 in]
              n33 = Close Reference(reference=w109, error in (no error)=w110) -> ()  [unwired: 1 out]
              n34 = Close Reference(reference=w108, error in (no error)=w107) -> ()  [unwired: 1 out]
              n35 = Or(x=w112, y=w113) -> (x .or. y?=w105:bool)
              n36 = Build Array(w79) -> (w77:dbl[])
              n37 = Build Array(w78) -> (w76:dbl[])
              n38 = Unbundle By Name(w84) -> ("Main Screen.zFF"=w103:refnum<vi>)
              n39 = Select(t=w77, s=w105, f=w76) -> (s? t:f=w104:dbl[])
              n40 = property class="Bool (strict)"(reference=w103) -> (reference out=w101:refnum<vi>, error out=w102:errorcluster, "Value"=w100:bool)  [unwired: 1 in]
              n41 = call-poly <vilib>:"Mean.vi"("X"=w104) -> ("mean"=w92:dbl)  [unwired: 1 out]
              n42 = Close Reference(reference=w101, error in (no error)=w102) -> ()  [unwired: 1 out]
              n43 = Unbundle By Name(w84) -> ("Config Parameters.SAMPLES"=w91:refnum<vi>)
              n44 = Unbundle By Name(w84) -> ("Config Parameters.Re-initilaize"=w93:refnum<vi>)
              n45 = Unbundle By Name(w84) -> ("Config Parameters.Filter ON/OFF"=w99:refnum<vi>)
              n46 = case shown="True" w100 {
                tunnel: w84 -> [_ w128]
                tunnel: w92 -> [_ w126]
                frame False {
                }
                frame True {
                  n47 = Unbundle By Name(w128) -> ("Main Screen.zFF"=w129:refnum<vi>)
                  n48 = property class="Bool (strict)"(reference=w129, "Value"=FALSE) -> (reference out=w131:refnum<vi>, error out=w130:errorcluster)  [unwired: 1 in]
                  n49 = Close Reference(reference=w131, error in (no error)=w130) -> ()  [unwired: 1 out]
                  "Fload" <- w126
                }
              }
              n50 = local read "Fload"() -> (w80:dbl)
              n51 = Subtract(x=w92, y=w80) -> (x-y=w81:dbl)
              "Friction" <- w81
              n52 = property class="Bool (strict)"(reference=w99) -> (reference out=w97:refnum<vi>, error out=w98:errorcluster, "Value"=w96:bool)  [unwired: 1 in]
              n53 = property class="DigNum (strict)"(reference=w91) -> (reference out=w89:refnum<vi>, error out=w90:errorcluster, "Value"=w88:dbl)  [unwired: 1 in]
              n54 = property class="Bool (strict)"(reference=w93) -> (reference out=w95:refnum<vi>, error out=w94:errorcluster, "Value"=w82:bool)  [unwired: 1 in]
              n55 = Close Reference(reference=w97, error in (no error)=w98) -> ()  [unwired: 1 out]
              n56 = Close Reference(reference=w95, error in (no error)=w94) -> ()  [unwired: 1 out]
              n57 = Close Reference(reference=w89, error in (no error)=w90) -> ()  [unwired: 1 out]
              n58 = case shown="True" w96 {
                tunnel: w82 -> [_ w120]
                tunnel: w84 -> [_ w119]
                tunnel: w81 -> [w114 w118]
                tunnel: w88 -> [_ w117]
                tunnel: [w114 w116] -> w83
                tunnel: w82 -> [_ w115]
                frame False {
                }
                frame True {
                  n59 = case shown="True" w115 {
                    tunnel: w119 -> [_ w122]
                    frame False {
                    }
                    frame True {
                      n60 = Unbundle By Name(w122) -> ("Config Parameters.Re-initilaize"=w125:refnum<vi>)
                      n61 = property class="Bool (strict)"(reference=w125, "Value"=FALSE) -> (reference out=w123:refnum<vi>, error out=w124:errorcluster)  [unwired: 1 in]
                      n62 = Close Reference(reference=w123, error in (no error)=w124) -> ()  [unwired: 1 out]
                    }
                  }
                  n63 = call <vilib>:"Mean PtByPt.vi"("x"=w118, "sample length"=w117, "initialize"=w120) -> ("mean"=w116:dbl)  [unwired: 1 in, 1 out]
                }
              }
              n64 = Unbundle By Name(w84) -> ("Main Screen.Friction Force (N)"=w85:refnum<vi>)
              n65 = property class="DigNum (strict)"(reference=w85, "Value"=w83) -> (reference out=w87:refnum<vi>, error out=w86:errorcluster)  [unwired: 1 in]
              n66 = Close Reference(reference=w87, error in (no error)=w86) -> ()  [unwired: 1 out]
            }
            frame True {
              n67 = Unbundle By Name(w138) -> ("Loading Com Port.FORCE (N)"=w166:refnum<vi>)
              n68 = property class="WFChart (strict)"(reference=w166) -> (reference out=w164:refnum<vi>, error out=w165:errorcluster, "History Data"=w135:dbl[][])  [unwired: 1 in]
              n69 = Unbundle By Name(w138) -> ("Main Screen.Friction Force (N)"=w154:refnum<vi>)
              n70 = Index Array(array=w135, index (col)=1 ("disabled index (col)")) -> (element=w134:dbl[])  [unwired: 1 in]
              n71 = Close Reference(reference=w164, error in (no error)=w165) -> ()  [unwired: 1 out]
              n72 = call-poly <vilib>:"Mean.vi"("X"=w134) -> ("mean"=w163:dbl)  [unwired: 1 out]
              n73 = Unbundle By Name(w138) -> ("Main Screen.CZ FF"=w145:refnum<vi>)
              n74 = Subtract(x=w134, y=w163) -> (x-y=w162:dbl[])
              n75 = property class="DigNum (strict)"(reference=w154) -> (reference out=w156:refnum<vi>, error out=w155:errorcluster, "Value"=w153:dbl)  [unwired: 1 in]
              n76 = property class="Bool (strict)"(reference=w145) -> (reference out=w143:refnum<vi>, error out=w144:errorcluster, "Value"=w142:bool)  [unwired: 1 in]
              n77 = call-poly <vilib>:"RMS.vi"("X"=w162) -> ("rms value"=w160:dbl)  [unwired: 1 out]
              n78 = Unbundle By Name(w138) -> ("Main Screen.zFF"=w152:refnum<vi>)
              n79 = Not A Number/Path/Refnum?(number/path/refnum=w160) -> (NaN/Path/Refnum?=w161:bool)
              n80 = Close Reference(reference=w156, error in (no error)=w155) -> ()  [unwired: 1 out]
              n81 = property class="Bool (strict)"(reference=w152) -> (reference out=w150:refnum<vi>, error out=w151:errorcluster, "Value"=w149:bool)  [unwired: 1 in]
              n82 = Close Reference(reference=w143, error in (no error)=w144) -> ()  [unwired: 1 out]
              n83 = Select(t=w153, s=w161, f=w160) -> (s? t:f=w148:dbl)
              n84 = case shown="True" w142 {
                tunnel: w138 -> [_ w169]
                tunnel: w132 -> [_ w167]
                frame False {
                }
                frame True {
                  n85 = Unbundle By Name(w169) -> ("Main Screen.CZ FF"=w170:refnum<vi>)
                  n86 = property class="Bool (strict)"(reference=w170, "Value"=FALSE) -> (reference out=w172:refnum<vi>, error out=w171:errorcluster)  [unwired: 1 in]
                  n87 = Close Reference(reference=w172, error in (no error)=w171) -> ()  [unwired: 1 out]
                  "Fload 3" <- w167
                }
              }
              n88 = Close Reference(reference=w150, error in (no error)=w151) -> ()  [unwired: 1 out]
              n89 = local read "Fload 2"() -> (w146:dbl)
              n90 = case shown="True" w149 {
                tunnel: w138 -> [_ w175]
                tunnel: w148 -> [_ w173]
                frame False {
                }
                frame True {
                  n91 = Unbundle By Name(w175) -> ("Main Screen.zFF"=w176:refnum<vi>)
                  n92 = property class="Bool (strict)"(reference=w176, "Value"=FALSE) -> (reference out=w178:refnum<vi>, error out=w177:errorcluster)  [unwired: 1 in]
                  n93 = Close Reference(reference=w178, error in (no error)=w177) -> ()  [unwired: 1 out]
                  "Fload 2" <- w173
                }
              }
              n94 = Unbundle By Name(w138) -> ("Main Screen.Friction Force (N)"=w157:refnum<vi>)
              n95 = local read "Fload 3"() -> (w141:dbl)
              n96 = Subtract(x=w148, y=w146) -> (x-y=w147:dbl)
              n97 = Subtract(x=w132, y=w141) -> (x-y=w136:dbl)
              n98 = property class="DigNum (strict)"(reference=w157, "Value"=w147) -> (reference out=w159:refnum<vi>, error out=w158:errorcluster)  [unwired: 1 in]
              n99 = Unbundle By Name(w138) -> ("Main Screen.Cyclic Friction Force (N)"=w139:refnum<vi>)
              n100 = Close Reference(reference=w159, error in (no error)=w158) -> ()  [unwired: 1 out]
              n101 = property class="DigNum (strict)"(reference=w139, "Value"=w136) -> (reference out=w137:refnum<vi>, error out=w140:errorcluster)  [unwired: 1 in]
              n102 = Close Reference(reference=w137, error in (no error)=w140) -> ()  [unwired: 1 out]
            }
          }
          n103 = call-poly <vilib>:"Mean.vi"("X"=w24) -> ("mean"=w73:dbl)  [unwired: 1 out]
          n104 = Negate(x=w73) -> (-x=w60:dbl)
          n105 = Unbundle By Name(w14) -> ("Main Screen.zNL 2"=w64:refnum<vi>)
          n106 = Unbundle By Name(w14) -> ("Motion Module.zNL"=w69:refnum<vi>)
          n107 = property class="Bool (strict)"(reference=w64) -> (reference out=w66:refnum<vi>, error out=w65:errorcluster, "Value"=w62:bool)  [unwired: 1 in]
          n108 = property class="Bool (strict)"(reference=w69) -> (reference out=w67:refnum<vi>, error out=w68:errorcluster, "Value"=w63:bool)  [unwired: 1 in]
          n109 = Close Reference(reference=w66, error in (no error)=w65) -> ()  [unwired: 1 out]
          n110 = Close Reference(reference=w67, error in (no error)=w68) -> ()  [unwired: 1 out]
          n111 = Or(x=w63, y=w62) -> (x .or. y?=w61:bool)
          n112 = case shown="True" w61 {
            tunnel: w60 -> [_ w202]
            tunnel: w14 -> [_ w195]
            frame False {
            }
            frame True {
              w194 = FALSE ("Value")
              n113 = Unbundle By Name(w195) -> ("Main Screen.zNL 2"=w196:refnum<vi>)
              n114 = Unbundle By Name(w195) -> ("Motion Module.zNL"=w201:refnum<vi>)
              n115 = property class="Bool (strict)"(reference=w196, "Value"=w194) -> (reference out=w198:refnum<vi>, error out=w197:errorcluster)  [unwired: 1 in]
              n116 = property class="Bool (strict)"(reference=w201, "Value"=w194) -> (reference out=w199:refnum<vi>, error out=w200:errorcluster)  [unwired: 1 in]
              n117 = Close Reference(reference=w198, error in (no error)=w197) -> ()  [unwired: 1 out]
              n118 = Close Reference(reference=w199, error in (no error)=w200) -> ()  [unwired: 1 out]
              "Zload" <- w202
            }
          }
          n119 = local read "Zload"() -> (w59:dbl)
          n120 = Subtract(x=w60, y=w59) -> (x-y=w54:dbl)
          n121 = Unbundle By Name(w14) -> ("PID.Vertical load (N)"=w72:refnum<vi>)
          n122 = Unbundle By Name(w14) -> ("Config Parameters.Apply Filter (Load)"=w56:refnum<vi>)
          n123 = property class="DigNum (strict)"(reference=w72, "Value"=w54) -> (reference out=w70:refnum<vi>, error out=w71:errorcluster)  [unwired: 1 in]
          n124 = property class="Bool (strict)"(reference=w56) -> (reference out=w58:refnum<vi>, error out=w57:errorcluster, "Value"=w55:bool)  [unwired: 1 in]
          n125 = Close Reference(reference=w70, error in (no error)=w71) -> ()  [unwired: 1 out]
          n126 = Close Reference(reference=w58, error in (no error)=w57) -> ()  [unwired: 1 out]
          n127 = case shown="True" w55 {
            tunnel: w14 -> [_ w190]
            tunnel: w54 -> [w179 w184]
            tunnel: [w179 w181] -> w51
            frame False {
            }
            frame True {
              n128 = Unbundle By Name(w190) -> ("Config Parameters.Filter%"=w193:refnum<vi>)
              n129 = property class="DigNum (strict)"(reference=w193) -> (reference out=w191:refnum<vi>, error out=w192:errorcluster, "Value"=w189:dbl)  [unwired: 1 in]
              n130 = Close Reference(reference=w191, error in (no error)=w192) -> ()  [unwired: 1 out]
              n131 = Multiply(x=w189, y=0.01) -> (x*y=w186:dbl)
              n132 = local read "Load Temp"() -> (w180:dbl)
              n133 = Subtract(x=1.0, y=w186) -> (x-y=w185:dbl)
              n134 = Multiply(x=w184, y=w185) -> (x*y=w183:dbl)
              n135 = Multiply(x=w186, y=w180) -> (x*y=w182:dbl)
              n136 = Add(x=w183, y=w182) -> (x+y=w181:dbl)
            }
          }
          n137 = Not A Number/Path/Refnum?(number/path/refnum=w51) -> (NaN/Path/Refnum?=w53:bool)
          n138 = Unbundle By Name(w14) -> ("Motion Module.NL disp"=w48:refnum<vi>)
          n139 = Unbundle By Name(w14) -> ("Main Screen.NL disp 2"=w47:refnum<vi>)
          n140 = Select(t=0.0, s=w53, f=w51) -> (s? t:f=w44:dbl)
          "Load Temp" <- w44
          n141 = property class="DigNum (strict)"(reference=w48, "Value"=w44) -> (reference out=w50:refnum<vi>, error out=w49:errorcluster)  [unwired: 1 in]
          n142 = property class="DigNum (strict)"(reference=w47, "Value"=w44) -> (reference out=w45:refnum<vi>, error out=w46:errorcluster)  [unwired: 1 in]
          n143 = Close Reference(reference=w50, error in (no error)=w49) -> ()  [unwired: 1 out]
          n144 = Close Reference(reference=w45, error in (no error)=w46) -> ()  [unwired: 1 out]
        }
      }
    }
    frame Error {
    }
  }
  "error out" <- w1
